vi "Create StringList.vi"(5 "StringList in":refnum<class "StringList.lvclass">, 7 "List Implementation (Array)":refnum<class "ListImp.lvclass">, 8 "error in (no error)":errorcluster) -> (0 "error out":errorcluster, 3 "StringList out":refnum<class "StringList.lvclass">)   [LabVIEW 2013, in "LapDog.Collections.v_.Lists.lvlib" / "StringList.lvclass"]
uses:
  StringList.lvclass
  ObjectList/ObjectList.lvclass
  ListImp/ListImp.lvclass
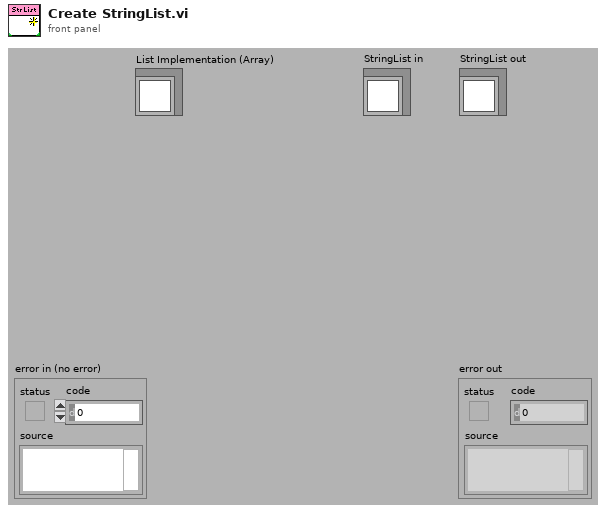
[diagram p1: front panel]
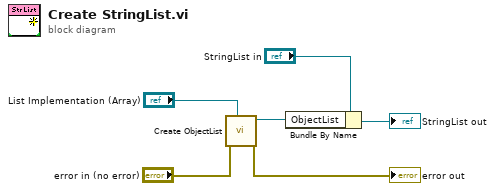
[diagram p0: block diagram]
diagram:
  n1 = call "Create ObjectList.vi"("List Implementation (Array)"="List Implementation (Array)", "error in (no error)"="error in (no error)") -> ("error out"=→"error out":errorcluster, "ObjectList"=w5:refnum<class "ObjectList.lvclass">)  [unwired: 8 in]
  n2 = Bundle By Name(cluster="StringList in", "ObjectList"=w5) -> (→"StringList out":refnum<class "StringList.lvclass">)
